vi "Get Profiles.vi"(8 "error in":errorcluster, 10 "OM  Location":T1) -> (0 "error out":errorcluster, 2 "folder names":string[](array[string]))   [LabVIEW 2013]
uses:
  Data Access Objects/Metadata/LBCB Location.ctl
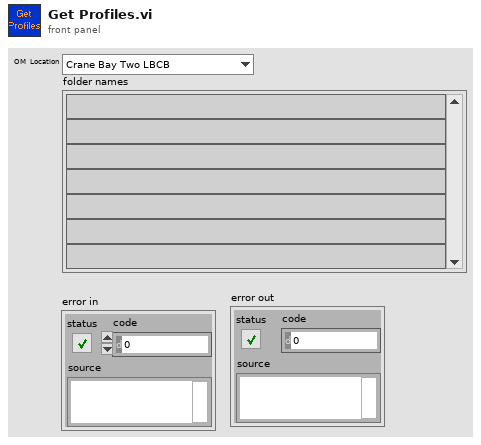
[diagram p1: front panel]
types:
  T1 = typedef "LBCB Location.ctl" = enum16{"Crane Bay Two LBCB", "Crane Bay One LBCB", "5th Scale Two LBCB", "5th Scale One LBCB", "Portable LBCB", "University of Houston LBCB"}
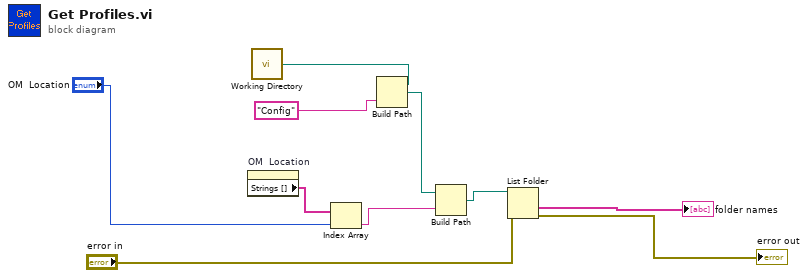
[diagram p0: block diagram]
diagram:
  n1 = property on="OM  Location" class="Enum (strict)"() -> ("Strings []"=w8:string[])  [unwired: 2 in, 2 out]
  n2 = call "Working Directory.vi"() -> ("Path"=w7:path)  [unwired: 1 out]
  n3 = Index Array(array=w8, index="OM  Location") -> (element=w9:string)
  n4 = Build Path(base path=w7, name or relative path="Config") -> (appended path=w10:path)
  n5 = Build Path(base path=w10, name or relative path=w9) -> (appended path=w4:path)
  n6 = List Folder(path=w4, error in="error in") -> (folder names=→"folder names":string[], error out=→"error out":errorcluster)  [unwired: 2 in, 2 out]
